vi "get-wnum.vi"() -> (0 "error out":errorcluster, 3 "wnum":dbl format="%#_9g")   [LabVIEW 2014]
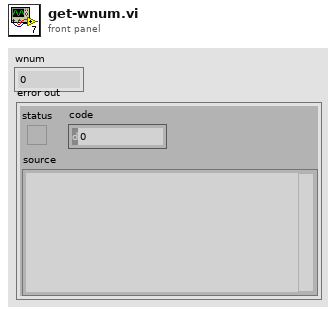
[diagram p1: front panel]
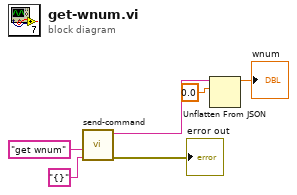
[diagram p0: block diagram]
diagram:
  n1 = call "send-command.vi"("parameters"="{}", "command"="get wnum") -> ("error out"=→"error out":errorcluster, "output"=w3:string)  [unwired: 8 in]
  n2 = Unflatten From JSON(JSON string=w3, type and defaults=0.0) -> (value=→"wnum":dbl)  [unwired: 5 in, 1 out]
